vi "WakerControl.vi"(6 "JS2 Button 4":bool, 7 "JS2 Button 1":bool, 8 "JS1 Button 4":bool, 9 "JS1 Button 1":bool) -> (2 "Speed Out":dbl)   [LabVIEW 2011]
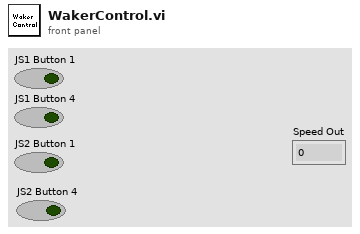
[diagram p1: front panel]
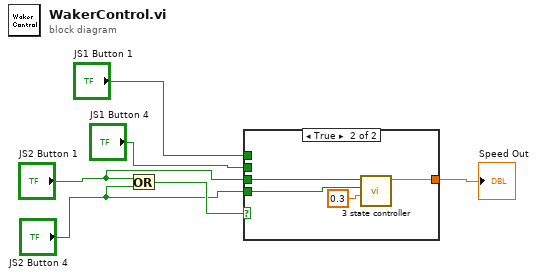
[diagram p0: block diagram]
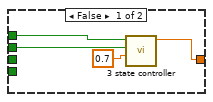
[diagram p2: hidden frame]
diagram:
  n1 = Or(x="JS2 Button 1", y="JS2 Button 4") -> (x .or. y?=w6:bool)
  n2 = case shown="True" w6 {
    tunnel: "JS2 Button 1" -> [_ w14]
    tunnel: "JS2 Button 4" -> [_ w13]
    tunnel: [w7 w11] -> w5
    tunnel: "JS1 Button 4" -> [w9 _]
    tunnel: "JS1 Button 1" -> [w10 _]
    frame False {
      n3 = call "3 state controller.vi"("Power"=0.7, "Backward"=w9, "Forward"=w10) -> ("Numeric"=w7:dbl)  [unwired: 8 in]
    }
    frame True {
      n4 = call "3 state controller.vi"("Power"=0.3, "Backward"=w13, "Forward"=w14) -> ("Numeric"=w11:dbl)  [unwired: 8 in]
    }
  }
  "Speed Out" <- w5
